vi "indice transposition.vi"(2 "error IN":errorcluster caption="error IO", 3 "indice entrée":string) -> (0 "error out":errorcluster caption="error IO", 1 "indice corrigé":string)   [LabVIEW 2020]
uses:
  Modules/FS/60_FS_Controles/60_FS_SetGet.ctl
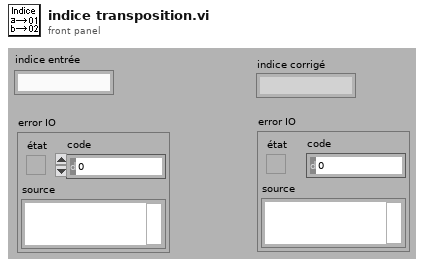
[diagram p1: front panel]
types:
  T1 = typedef "60_FS_SetGet.ctl" = enum16{"set", "get"}
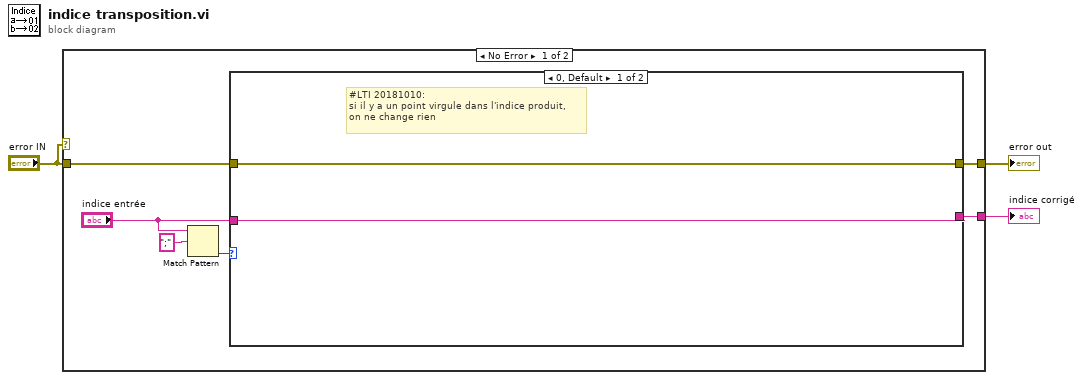
[diagram p0: block diagram]
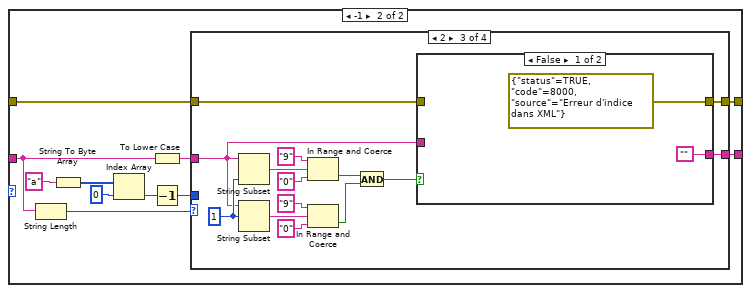
[diagram p2: hidden frame]
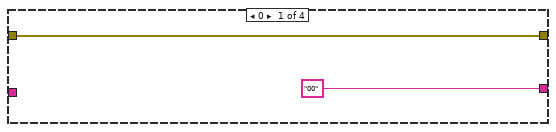
[diagram p3: hidden frame]
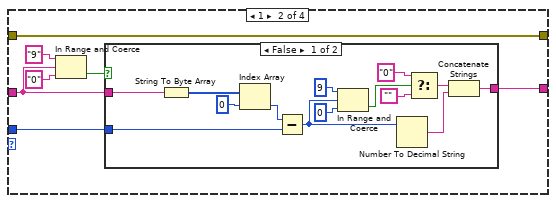
[diagram p4: hidden frame]
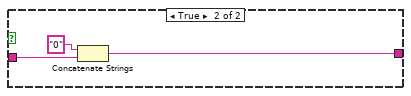
[diagram p5: hidden frame]
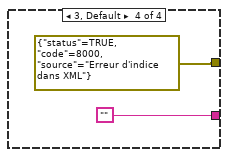
[diagram p7: hidden frame]
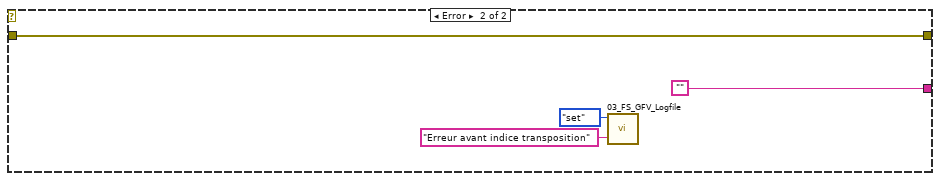
[diagram p8: hidden frame]
diagram:
  n1 = case shown="No Error" "error IN" {
    tunnel: [w9 w72] -> w3
    tunnel: [w8 ""] -> w2
    tunnel: "error IN" -> [w7 w72]
    frame No Error {
      n2 = Match Pattern(string="indice entrée", regular expression=";" ("expression régulière")) -> (offset past match=w4:i32)  [unwired: 1 in, 3 out]
      n3 = case shown="0, Default" w4 {
        tunnel: [w10 w15] -> w9
        tunnel: [w11 w14] -> w8
        tunnel: w7 -> [w10 w13]
        tunnel: "indice entrée" -> [w11 w12]
        frame 0, Default {
          # "#LTI 20181010:\nsi il y a un point virgule dans l'indice produit,\non ne change rien"
        }
        frame -1 {
          n4 = String Length(string=w12) -> (length=w18:i32)
          n5 = String To Byte Array(string="a" ("chaîne")) -> (unsigned byte array=w21:u8[])
          n6 = Index Array(array=w21, index=0 ("indice")) -> (element=w19:u8)
          n7 = To Lower Case(string=w12) -> (all lower case string=w17:string)
          n8 = Decrement(x=w19) -> (x-1=w16:u8)
          n9 = case shown="2" w18 {
            tunnel: [w24 w31 w51 errorcluster {"status"=TRUE, "code"=8000, "source"="Erreur d'indice dans XML"} ("error IO")] -> w15
            tunnel: w13 -> [w24 w31 w52 _]
            tunnel: ["00" w30 w50 ""] -> w14
            tunnel: w17 -> [_ w28 w49 _]
            tunnel: w16 -> [_ w29 _ _]
            frame 0 {
            }
            frame 1 {
              n10 = In Range and Coerce(upper limit="9" ("limite supérieure"), x=w28, lower limit="0" ("limite inférieure")) -> (In Range?=w25:bool)  [unwired: 1 out]
              n11 = case shown="False" w25 {
                tunnel: [w37 w46] -> w30
                tunnel: w29 -> [w42 _]
                tunnel: w28 -> [w41 w48]
                frame False {
                  n12 = String To Byte Array(string=w41) -> (unsigned byte array=w45:u8[])
                  n13 = Index Array(array=w45, index=0 ("indice")) -> (element=w43:u8)
                  n14 = Subtract(x=w43, y=w42) -> (x-y=w40:u8)
                  n15 = In Range and Coerce(upper limit=u8 9 ("limite supérieure"), x=w40, lower limit=u8 0 ("limite inférieure")) -> (In Range?=w34:bool)  [unwired: 1 out]
                  n16 = Number To Decimal String(number=w40) -> (decimal integer string=w36:string)  [unwired: 1 in]
                  n17 = Select(t="0" ("limite inférieure"), s=w34, f="") -> (s? t:f=w35:string)
                  n18 = Concatenate Strings(w35, w36) -> (w37:string)
                }
                frame True {
                  n19 = Concatenate Strings("0" ("chaîne"), w48) -> (w46:string)
                }
              }
            }
            frame 2 {
              w60 = 1 ("longueur (reste)")
              n20 = String Subset(string=w49, length (rest)=w60) -> (substring=w57:string)  [unwired: 1 in]
              n21 = String Subset(string=w49, offset (0)=w60) -> (substring=w56:string)  [unwired: 1 in]
              n22 = In Range and Coerce(upper limit="9" ("limite supérieure"), x=w57, lower limit="0" ("limite inférieure")) -> (In Range?=w54:bool)  [unwired: 1 out]
              n23 = In Range and Coerce(upper limit="9" ("limite supérieure"), x=w56, lower limit="0" ("limite inférieure")) -> (In Range?=w53:bool)  [unwired: 1 out]
              n24 = And(x=w54, y=w53) -> (x .and. y?=w55:bool)
              n25 = case shown="False" w55 {
                tunnel: w52 -> [_ w66]
                tunnel: [errorcluster {"status"=TRUE, "code"=8000, "source"="Erreur d'indice dans XML"} ("error IO") w66] -> w51
                tunnel: ["" w65] -> w50
                tunnel: w49 -> [_ w65]
                frame False {
                }
                frame True {
                }
              }
            }
            frame 3, Default {
            }
          }
        }
      }
    }
    frame Error {
      n26 = call "03_FS_GFV_Logfile.vi"("Chaîne"="Erreur avant indice transposition", "States"=60_FS_SetGet."set") -> ()  [unwired: 8 in, 2 out]
    }
  }
  "error out" <- w3
  "indice corrigé" <- w2
